vi "Andy.vi"   [LabVIEW 2016]
uses:
  <vilib>/NXT/Block Support/NXT_OutputPort.ctl
  <vilib>/NXT/Block Support/NXT_InputPort.ctl
  <vilib>/NXT/Dual Mode Library/Sensors/Light_On.vi
  <vilib>/NXT/NXTIO Xnodes/NXTIONodeSubVIs/NXTMoveMotors.vi
  <vilib>/NXT/Dual Mode Library/Sensors/Sonar_cm.vi
  <vilib>/NXT/Dual Mode Library/Display/drawNumber_float.vi
  <vilib>/NXT/NXTIO Xnodes/NXTIONodeSubVIs/NXTStopMotors.vi
  <vilib>/NXT/Dual Mode Library/Waits/Wait_Rotation.vi
  <vilib>/NXT/NXTIO Xnodes/NXTIONodeSubVIs/NXTMotorRunDistance.vi
  <vilib>/NXT/NXTIO Xnodes/AddressXNode/NXTIOAddress.xnode
  <vilib>/NXT/NXTIO Xnodes/NXTIOXNode/NXTIO.xnode
  <vilib>/NXT/Subs/LVHSConnector.ctl
  <vilib>/NXT/LegoClasses/BrickReference/BrickReference.lvclass
types:
  T1 = typedef "NXT_OutputPort.ctl" = u8
  T2 = typedef "NXT_InputPort.ctl" = u32
  T3 = typedef "LVHSConnector.ctl" = refnum<class "BrickReference.lvclass">
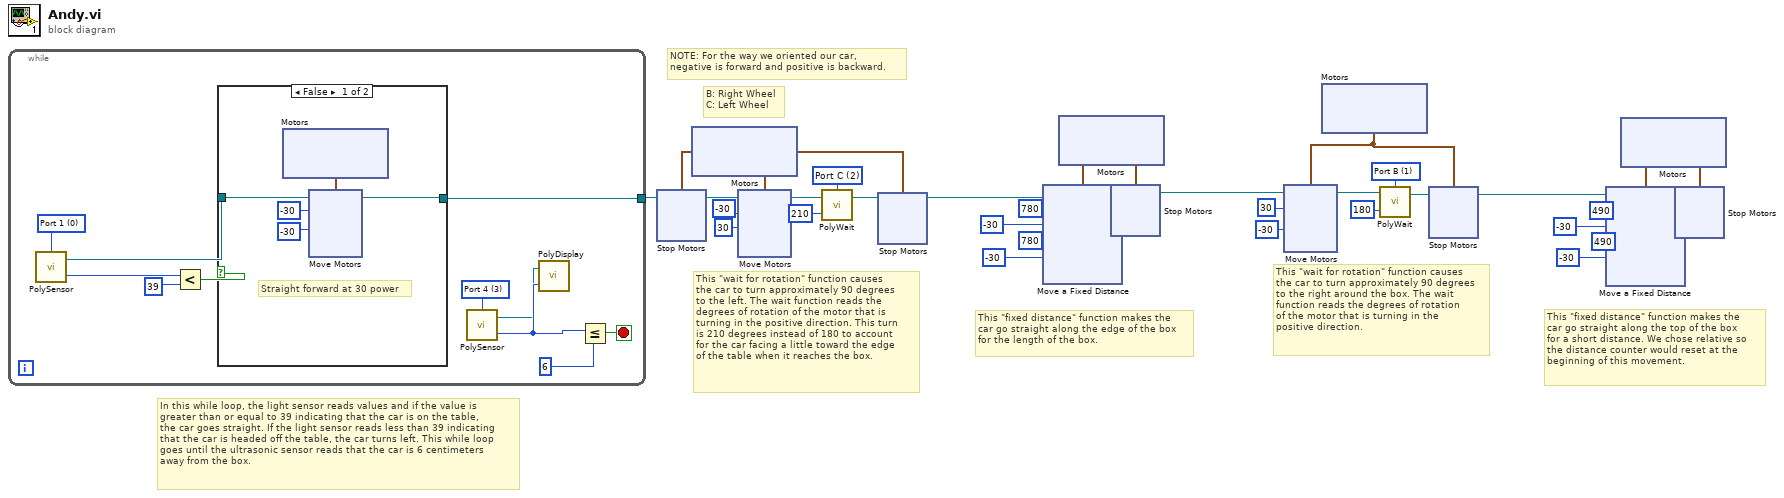
[diagram p0: block diagram]
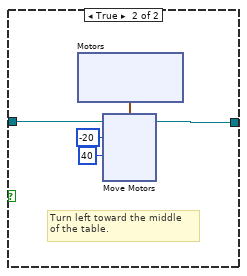
[diagram p2: hidden frame]
diagram:
  w15 = T1 1 items=["Port A", "Port B", "Port C", "Port D"] ("Port (Port A)")
  w28 = T1 2 items=["Port A", "Port B", "Port C", "Port D"] ("Port (Port A)")
  # "NOTE: For the way we oriented our car,\nnegative is forward and positive is backward."
  # "B: Right Wheel\nC: Left Wheel"
  # "This \"fixed distance\" function makes the\ncar go straight along the top of the box\nfor a short distance. We chose relative so \nthe distance counter would reset at the\nbeginning of this movement."
  # "This \"wait for rotation\" function causes\nthe car to turn approximately 90 degrees\nto the right around the box. The wait \nfunction reads the degrees of rotation \nof the motor that is turning in the \npositive direction."
  # "This \"fixed distance\" function makes the\ncar go straight along the edge of the box\nfor the length of the box."
  # "This \"wait for rotation\" function causes\nthe car to turn approximately 90 degrees\nto the left. The wait function reads the \ndegrees of rotation of the motor that is\nturning in the positive direction. This turn \nis 210 degrees instead of 180 to account \nfor the car facing a little toward the edge \nof the table when it reaches the box."
  # "In this while loop, the light sensor reads values and if the value is \ngreater than or equal to 39 indicating that the car is on the table, \nthe car goes straight. If the light sensor reads less than 39 indicating \nthat the car is headed off the table, the car turns left. This while loop\ngoes until the ultrasonic sensor reads that the car is 6 centimeters \naway from the box."
  n1 = while {
    tunnel: [w37] -> w3
    stop <- w34 stop-if-true
    w36 = T2 3 items=["Port 1", "Port 2", "Port 3", "Port 4"] ("Port (Port 4)")
    w42 = T2 0 items=["Port 1", "Port 2", "Port 3", "Port 4"] ("Port (Port 4)")
    n2 = call-poly <vilib>:"PolySensor.vi"("Port (Port 3)"=w42) -> ("Scaled Value"=w40:i16, "NXT/EV3"=w38:T3)  [unwired: 2 in]
    n3 = Less?(x=w40, y=i16 39) -> (x < y?=w41:bool)
    n4 = case shown="False" w41 {
      tunnel: w38 -> [w44 w60]
      tunnel: [w43 w57] -> w37
      frame False {
        # "Straight forward at 30 power"
        n5 = xnode "Motors"() -> ("Motor"=w47:cluster{"Port":T1, "Port":T1})
        n6 = xnode "Move Motors"("Power/Speed 1"=i8 -30, "Motors"=w47, "NXT/EV3"=w44, "Power/Speed 2"=i8 -30) -> ("NXT/EV3"=w43:T3)
      }
      frame True {
        # "Turn left toward the middle \nof the table."
        n7 = xnode "Motors"() -> ("Motor"=w61:cluster{"Port":T1, "Port":T1})
        n8 = xnode "Move Motors"("Power/Speed 2"=i8 40, "Power/Speed 1"=i8 -20, "Motors"=w61, "NXT/EV3"=w60) -> ("NXT/EV3"=w57:T3)
      }
    }
    n9 = call-poly <vilib>:"PolySensor.vi"("Port (Port 4)"=w36) -> ("Distance (cm)"=w33:i16, "NXT/EV3"=w32:T3)  [unwired: 2 in]
    n10 = call-poly <vilib>:"PolyDisplay.vi"("number"=w33, "NXT/EV3"=w32) -> ()  [unwired: 2 in, 1 out]
    n11 = Less Or Equal?(x=w33, y=i16 6) -> (x <= y?=w34:bool)
  }
  n12 = xnode "Motors"() -> ("Motor"=w1:cluster{"Port":T1, "Port":T1})
  n13 = xnode "Stop Motors"("Motors"=w1, "NXT/EV3"=w3) -> ("NXT/EV3"=w2:T3)
  n14 = xnode "Move Motors"("Power/Speed 1"=-30 ("Steering 1"), "Motors"=w1, "NXT/EV3"=w2, "Power/Speed 2"=i8 30 ("Power/Speed 1")) -> ("NXT/EV3"=w29:T3)
  n15 = call-poly <vilib>:"PolyWait.vi"("Position Change (180)"=210, "NXT/EV3"=w29, "Port (Port A)"=w28) -> ("NXT/EV3"=w26:T3)  [unwired: 1 in]
  n16 = xnode "Stop Motors"("Motors"=w1, "NXT/EV3"=w26) -> ("NXT/EV3"=w21:T3)
  n17 = xnode "Motors"() -> ("Motor"=w22:cluster{"Port":T1, "Port":T1})
  n18 = xnode "Move a Fixed Distance"("Speed 2"=i8 -30 ("Power/Speed 2"), "Speed 1"=i8 -30 ("Power/Speed 1"), "Distance 2"=780, "Distance 1"=780, "Motors"=w22, "NXT/EV3"=w21) -> ("NXT/EV3"=w23:T3)
  n19 = xnode "Stop Motors"("Motors"=w22, "NXT/EV3"=w23) -> ("NXT/EV3"=w11:T3)
  n20 = xnode "Motors"() -> ("Motor"=w12:cluster{"Port":T1, "Port":T1})
  n21 = xnode "Move Motors"("Power/Speed 1"=30 ("Steering 1"), "Motors"=w12, "NXT/EV3"=w11, "Power/Speed 2"=i8 -30 ("Power/Speed 1")) -> ("NXT/EV3"=w16:T3)
  n22 = call-poly <vilib>:"PolyWait.vi"("Position Change (180)"=180, "NXT/EV3"=w16, "Port (Port A)"=w15) -> ("NXT/EV3"=w13:T3)  [unwired: 1 in]
  n23 = xnode "Stop Motors"("Motors"=w12, "NXT/EV3"=w13) -> ("NXT/EV3"=w6:T3)
  n24 = xnode "Motors"() -> ("Motor"=w5:cluster{"Port":T1, "Port":T1})
  n25 = xnode "Move a Fixed Distance"("Speed 2"=i8 -30 ("Power/Speed 2"), "Speed 1"=i8 -30 ("Power/Speed 1"), "Distance 2"=490, "Distance 1"=490, "Motors"=w5, "NXT/EV3"=w6) -> ("NXT/EV3"=w4:T3)
  n26 = xnode "Stop Motors"("Motors"=w5, "NXT/EV3"=w4) -> ()  [unwired: 1 out]
